vi "VI, Get Panel Width.vi"(6 "error in":errorcluster, 9 "VI ref":refnum<vi>) -> (0 "error out":errorcluster, 3 "VI ref dup":refnum<vi>, 4 "width":i16=20)   [LabVIEW 2010]
doc: "This function gets a front panel width in pixel units."
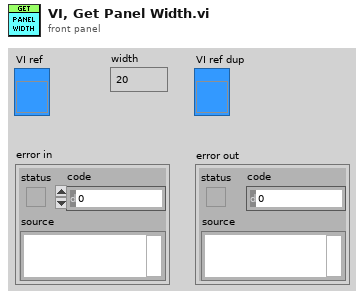
[diagram p1: front panel]
types:
  T1 = typedef "LVRectTypeDef.ctl" = cluster{"left":i16, "top":i16, "right":i16, "bottom":i16}
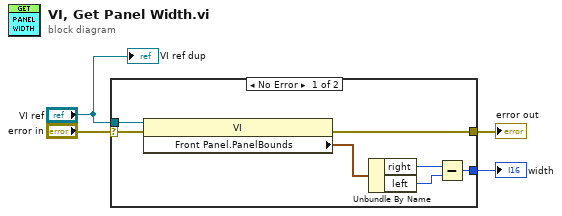
[diagram p0: block diagram]
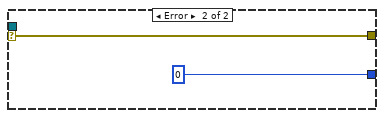
[diagram p2: hidden frame]
diagram:
  n1 = case shown="No Error" "error in" {
    selector: "error in" -> [w10 w13]
    tunnel: "VI ref" -> [w11 _]
    tunnel: [w9 w13] -> w4
    tunnel: [w6 i16 0] -> w1
    frame No Error {
      n2 = property class="VI"(reference=w11, error in=w10) -> (error out=w9:errorcluster, "Front Panel.PanelBounds"=w5:T1)  [unwired: 1 out]
      n3 = Unbundle By Name(w5) -> ("right"=w8:i16, "left"=w7:i16)
      n4 = Subtract(x=w8, y=w7) -> (x-y=w6:i16)
    }
    frame Error {
    }
  }
  "error out" <- w4
  "width" <- w1
  "VI ref dup" <- "VI ref"
